vi "Read PlatMods.vi"(8 "error in (no error)":errorcluster, 11 "ControlMouseUpMsg in":refnum<class "ControlMouseUpMsg.lvclass">) -> (0 "error out":errorcluster, 2 "PlatMods":T1, 3 "ControlMouseUpMsg out":refnum<class "ControlMouseUpMsg.lvclass">)   [LabVIEW 2017, in "ActorEvents.lvlib" / "ControlMouseUpMsg.lvclass"]
uses:
  ControlMouseUpMsg.lvclass
  ControlMouseUpMsg.lvclass/ControlMouseUpMsg.ctl
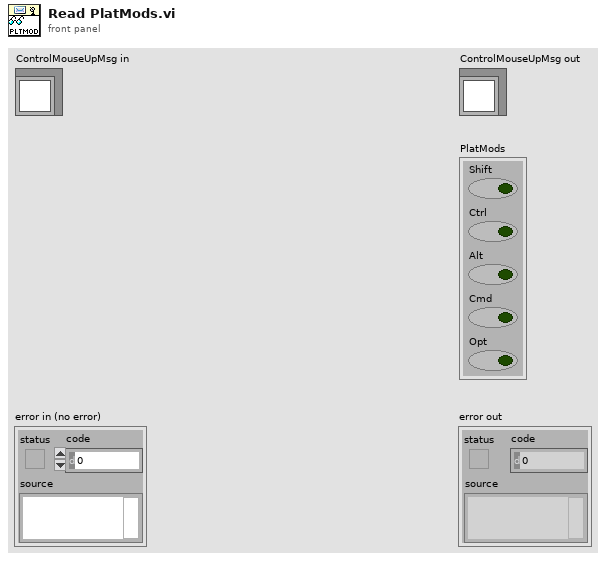
[diagram p1: front panel]
types:
  T1 = cluster{"Shift":bool, "Ctrl":bool, "Alt":bool, "Cmd":bool, "Opt":bool}
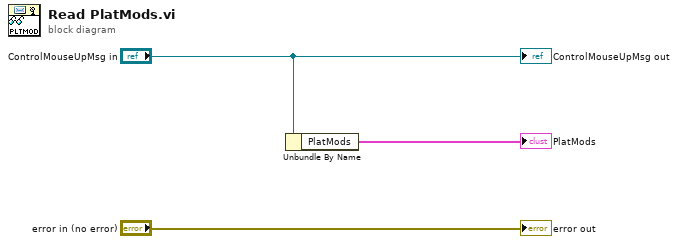
[diagram p0: block diagram]
diagram:
  n1 = Unbundle By Name("ControlMouseUpMsg in") -> ("PlatMods"=→"PlatMods":T1)
  "error out" <- "error in (no error)"
  "ControlMouseUpMsg out" <- "ControlMouseUpMsg in"
